vi "ROE200_DriverUse.vi"(0 "VISA resource name In":refnum<visa-resource-name>, 1 "CMD":T1(ring), 5 "X":u32, 7 "Y":u32, 9 "Z":u32, 11 "error in":errorcluster) -> (4 "VISA resource name out":refnum<visa-resource-name>, 6 "X 2":u32, 8 "Y 2":u32, 10 "Z 2":u32, 15 "error out":errorcluster)   [LabVIEW 2019]
panel:
  in  "E Stop":bool
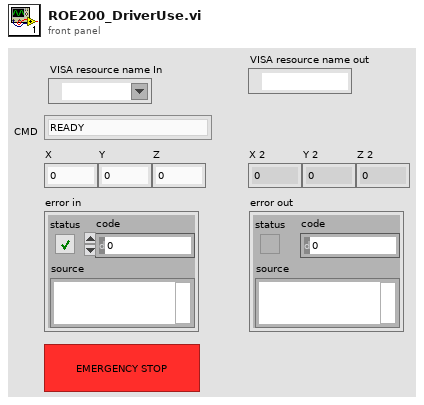
[diagram p1: front panel]
types:
  T1 = enum16{"READY", "ABSOLUTE MOVE", "RELATIVE MOVE", "HOMING", "WAITING", "CANCELING"}
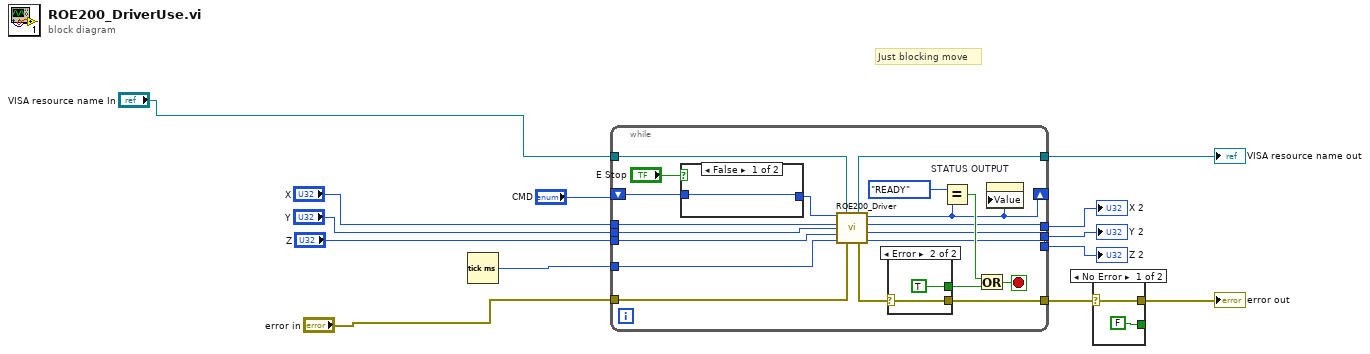
[diagram p0: block diagram]
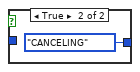
[diagram p2: hidden frame]
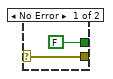
[diagram p3: hidden frame]
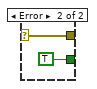
[diagram p4: hidden frame]
diagram:
  # "Just blocking move"
  n1 = Tick Count (ms)() -> (millisecond timer value=w7:u32)
  n2 = while {
    tunnel: "VISA resource name In" -> [w26]
    shift-right: [w14] -> _
    shift-left: "CMD" -> [w27]
    tunnel: [w25] -> w13
    tunnel: [w30] -> w8
    tunnel: "error in" -> [w19]
    tunnel: [w17] -> w6
    tunnel: [w16] -> w5
    tunnel: [w15] -> w4
    tunnel: "X" -> [w23]
    tunnel: "Y" -> [w22]
    tunnel: "Z" -> [w21]
    tunnel: w7 -> [w20]
    stop <- w33 stop-if-true
    n3 = case shown="False" "E Stop" {
      tunnel: w27 -> [w34 _]
      tunnel: [w34 T1."CANCELING" ("STATUS INPUT")] -> w24
      frame False {
      }
      frame True {
      }
    }
    n4 = call "ROE200_Driver.vi"("STATUS INPUT"=w24, "VISA resource name"=w26, "X 2"=w23, "Y 2"=w22, "Z 2"=w21, "Timing"=w20, "error in (no error) 2"=w19) -> ("VISA resource name out"=w25:refnum<visa-resource-name>, "STATUS OUTPUT"=w14:T1, "X Position"=w17:u32, "Y Position"=w16:u32, "error out 2"=w18:errorcluster, "Z Position"=w15:u32)  [unwired: 3 in]
    n5 = case shown="Error" w18 {
      selector: w18 -> [w36 w38]
      tunnel: [FALSE TRUE] -> w31
      tunnel: [w36 w38] -> w30
      frame No Error {
      }
      frame Error {
      }
    }
    n6 = Equal?(x=T1."READY" ("STATUS OUTPUT"), y=w14) -> (x = y?=w32:bool)
    n7 = Or(x=w32, y=w31) -> (x .or. y?=w33:bool)
    n8 = property on="STATUS OUTPUT" class="Enum (strict)"("Value"=w14) -> ()  [unwired: 2 in, 2 out]
  }
  "VISA resource name out" <- w13
  "X 2" <- w6
  "Y 2" <- w5
  "Z 2" <- w4
  n9 = case shown="No Error" w8 {
    selector: w8 -> [w40 w43]
    tunnel: [FALSE TRUE] -> _
    tunnel: [w40 w43] -> w12
    frame No Error {
    }
    frame Error {
    }
  }
  "error out" <- w12
